vi "BEEPERCALIBRATION.vi"() -> ()   [LabVIEW 2014]
panel:
  out "fundamental frequency":dbl format="%.2p"
  out "CAL FACTOR":dbl
  in  "TONE GENERATOR AMPLITUDE":dbl=94.0
  out "fundamental dB output":dbl
  out "PASS/FAIL 4":bool caption="CAL STATUS"
  out "N Harmonics":i32
  in  "offset":dbl=137.0
  # "BEEPER CALIBRATION"
  # "INPUT VALUE"
  # "OUTPUT VALUE"
  # "[RED = INPROCESS; GREEN = COMPLETE"
  # "OUTPUT VALUE"
  # "OUTPUT VALUE"
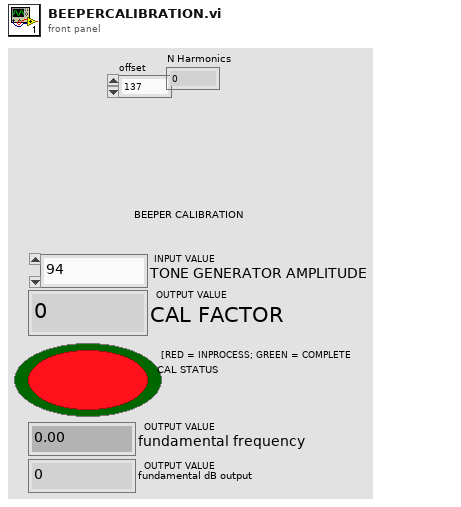
[diagram p1: front panel]
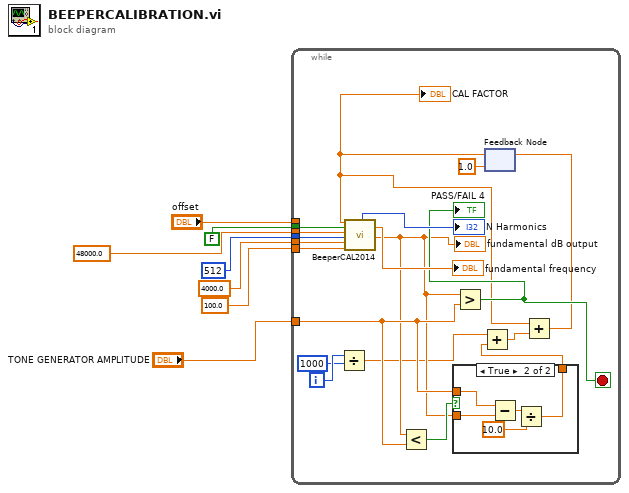
[diagram p0: block diagram]
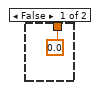
[diagram p2: hidden frame]
diagram:
  n1 = while {
    tunnel: "offset" -> [_]
    tunnel: FALSE ("Init") -> [w26]
    tunnel: 48000.0 ("sample rate") -> [w25]
    tunnel: 512 ("number of samples") -> [w24]
    tunnel: 4000.0 ("Upper Cut-Off") -> [w23]
    tunnel: 100.0 ("Lower Cut-Off") -> [w22]
    tunnel: "TONE GENERATOR AMPLITUDE" -> [w15]
    i -> [w19]
    stop <- w17 stop-if-true
    n2 = Divide(x=w19, y=1000) -> (x/y=w12:dbl)
    n3 = feedback #1(1.0) -> (w8:dbl)
    "CAL FACTOR" <- w8
    n4 = call "BeeperCAL2014.VI"("offset"=w8, "Init"=w26, "sample rate"=w25, "number of samples"=w24, "Upper Cut-Off"=w23, "Lower Cut-Off"=w22) -> ("N Harmonics"=→"N Harmonics":i32, "fundamental frequency"=→"fundamental frequency":dbl, "fundamental dB output"=w14:dbl)  [unwired: 6 in, 5 out]
    "fundamental dB output" <- w14
    n5 = Less?(x=w14, y=w15) -> (x < y?=w16:bool)
    n6 = case shown="True" w16 {
      tunnel: w15 -> [_ w32]
      tunnel: w14 -> [_ w31]
      tunnel: [0.0 w28] -> w13
      frame False {
      }
      frame True {
        n7 = Subtract(x=w32, y=w31) -> (x-y=w30:dbl)
        n8 = Divide(x=w30, y=10.0) -> (x/y=w28:dbl)
      }
    }
    n9 = Greater?(x=w14, y=w15) -> (0:w17:bool)
    "PASS/FAIL 4" <- w17
    n10 = Add(x=w12, y=w13) -> (x+y=w10:dbl)
    n11 = Add(x=w8, y=w10) -> (x+y=w9:dbl)
    n12 = feedback-in #1(w9) -> ()
  }
